vi "Add New MetaData Array.vi"(8 "error in (no error)":errorcluster, 11 "Node Ptr":u64 format="%.0x") -> (0 "error out":errorcluster)   [LabVIEW 2013, in "Instrument Addon System Explorer.lvlib"]
uses:
  Instrument Addon System Explorer.lvlib
  Shared/Types/FG Control.ctl
  Shared/Types/MetaData Parameters.ctl
  Shared/Types/Protocol Data Type.ctl
  Shared/Types/Metadata Channel Type.ctl
  Shared/Types/Type Cast Type.ctl
  Shared/Constants.vi
  <vilib>/NI Veristand/Custom Device API/Set Item Property (String).vi
  <vilib>/NI Veristand/Custom Device API/Set Item Property (Variant).vi
  <vilib>/NI Veristand/Custom Device API/Custom Device API.lvlib
  Shared/Instrument Addon Shared.lvlib
panel:
  in  "Tag":string
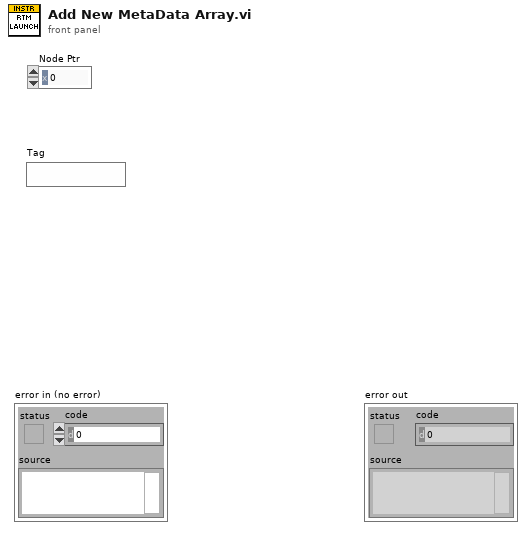
[diagram p1: front panel]
types:
  T1 = typedef "Instrument Addon Shared.lvlib/MetaData Parameters.ctl" = cluster{"Data Type":T2, "Channel Type":T3, "List":string[], "Format String":string, "Type":T4, "Delimiter":string}
  T2 = typedef "Instrument Addon Shared.lvlib/Protocol Data Type.ctl" = enum16{"Single Channel", "Array"}
  T3 = typedef "Instrument Addon Shared.lvlib/Metadata Channel Type.ctl" = enum16{"Enumerated List", "Format", "Type Cast"}
  T4 = typedef "Instrument Addon Shared.lvlib/Type Cast Type.ctl" = enum16{"DBL", "SGL", "U64", "U32", "U16", "U8", "I64", "I32", "I16", "I8"}
  T5 = typedef "Instrument Addon Shared.lvlib/FG Control.ctl" = enum16{"Get", "Set"}
  T6 = typedef "Custom Device API.lvlib/Custom Device Item Info.ctl" = cluster{"Name":string, "Is Channel":bool, "GUID":string, "Is Waveform":bool}
  T7 = typedef "Custom Device API.lvlib/Custom Device Item Ref.ctl" = u64
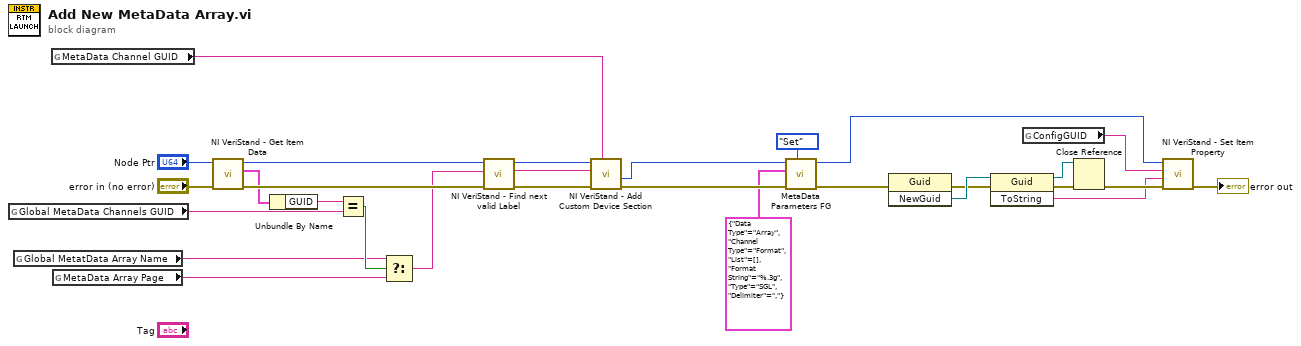
[diagram p0: block diagram]
diagram:
  n1 = global read "Constants.vi" "Global MetaData Channels GUID"() -> (w19:string)
  n2 = global read "Constants.vi" "Global MetatData Array Name"() -> (w17:string)
  n3 = global read "Constants.vi" "MetaData Channel GUID"() -> (w26:string)
  n4 = global read "Constants.vi" "MetaData Array Page"() -> (w16:string)
  n5 = call <vilib>:"NI VeriStand - Get Item Data.vi"("error in (no error)"="error in (no error)", "Item Ref in"="Node Ptr") -> ("error out"=w24:errorcluster, "Item Info"=w21:T6, "Item Ref out"=w22:T7)  [unwired: 6 in, 1 out]
  n6 = Unbundle By Name(w21) -> ("GUID"=w20:string)
  n7 = Equal?(x=w20, y=w19) -> (x = y?=w18:bool)
  n8 = Select(t=w17, s=w18, f=w16) -> (s? t:f=w15:string)
  n9 = call <vilib>:"NI VeriStand - Find next valid Label.vi"("error in (no error)"=w24, "Label"=w15, "Item Ref in"=w22) -> ("error out"=w27:errorcluster, "Label out"=w28:string, "Item Ref out"=w29:T7)  [unwired: 4 in, 2 out]
  n10 = call <vilib>:"NI VeriStand - Add Custom Device Section.vi"("GUID (Default Section)"=w26, "error in (no error)"=w27, "Section Name"=w28, "Parent Ref in"=w29) -> ("error out"=w5:errorcluster, "Section Ptr"=w3:T7)  [unwired: 4 in, 2 out]
  n11 = call "MetaData Parameters FG.vi"("Action"=FG_Control."Set", "error in (no error)"=w5, "MetaData Parameters"=T1 {"Data Type"=enum."Array", "Channel Type"=enum."Format", "List"=[], "Format String"="%.3g", "Type"=enum."SGL", "Delimiter"=","}, "Item Ref in"=w3) -> ("error out"=w4:errorcluster, "Item Ref out"=w2:T7)  [unwired: 5 in, 1 out]
  n12 = invoke class="Guid" method="NewGuid"(error in=w4) -> (error out=w10:errorcluster, "NewGuid"=w11:refnum<k24>)  [unwired: 2 in, 1 out]
  n13 = invoke class="Guid" method="ToString"(reference=w11, error in=w10) -> (reference out=w12:refnum<k24>, error out=w9:errorcluster, "ToString"=w7:string)  [unwired: 1 in]
  n14 = global read "Constants.vi" "ConfigGUID"() -> (w14:string)
  n15 = Close Reference(reference=w12, error in (no error)=w9) -> (error out=w8:errorcluster)
  n16 = call-poly <vilib>:"NI VeriStand - Set Item Property.vi"("error in (no error)"=w8, "Value"=w7, "Property Name"=w14, "Item Ref in"=w2) -> ("error out"=→"error out":errorcluster)  [unwired: 5 in, 2 out]
